vi "Auto State Machine.vi"   [LabVIEW 2013]
uses:
  typedefs/fg_typedef.ctl
  typedefs/State Machine/singleUseSubstate.ctl
  typedefs/State Machine/subStates.ctl
  typedefs/DevRef Type.ctl
  typedefs/Vision/vision enable.ctl
panel:
  # "A State Machine to Handle One or Two Ball Autonomous"
types:
  T1 = typedef "fg_typedef.ctl" = enum16{"Get", "Set"}
  T2 = typedef "subStates.ctl" = enum16{"null", "wait", "driver control", "auto", "manual override", "hold position", "rotate", "pickup", "pass", "recover pass", "load", "goto shoot", "shoot high goal", "shoot low goal", "cancel arm", "cancel shooter", "end", "test"}
  T3 = typedef "singleUseSubstate.ctl" = enum16{"null", "wait", "shift high", "shift low", "extend shooter", "retract shooter", "latch", "unlatch", "end"}
  T4 = typedef "vision enable.ctl" = enum16{"Enable", "Disable", "Stop"}
  T5 = typedef "DevRef Type.ctl" = enum16{"Shooter Solenoid", "Latch Solenoid", "Right Up Sensor", "Right Down Sensor", "Hold Sensor", "Arm Encoder"}
  T6 = typedef "WPI_EncoderDevRef.ctl" = cluster{"DevStatus":errorcluster, "EncoderIndex":T7, "CounterIndex":T8, "DistancePerCount":dbl, "Decoding Type":T9}
  T7 = typedef "FPGA_EncoderIdx.ctl" = enum8{"Enc 0", "Enc 1", "Enc 2", "Enc 3", "Invalid"}
  T8 = typedef "FPGA_CounterCtrSystemIndex.ctl" = enum8{"Ctr 0", "Ctr 1", "Ctr 2", "Ctr 3", "Ctr 4", "Ctr 5", "Ctr 6", "Ctr 7", "Invalid"}
  T9 = typedef "WPI_EncoderType.ctl" = enum16{"1x", "2x", "4x"}
  T10 = typedef "vision data.ctl" = cluster{"x":dbl, "y":dbl, "area":dbl, "width":dbl, "height":dbl, "Hot Goal Present?":bool, "distance":dbl}
  T11 = typedef "WPI_DigitalInputDevRef.ctl" = cluster{"DevStatus":errorcluster, "DIO Channel":T12, "Digital Module":T13}
  T12 = typedef "FPGA_DIOChannel.ctl" = enum8{"DIO 1", "DIO 2", "DIO 3", "DIO 4", "DIO 5", "DIO 6", "DIO 7", "DIO 8", "DIO 9", "DIO 10", "DIO 11", "DIO 12", "DIO 13", "DIO 14", "Invalid"}
  T13 = typedef "FPGA_TypedefDigitalModule.ctl" = enum16{"Digital Module 1", "Digital Module 2"}
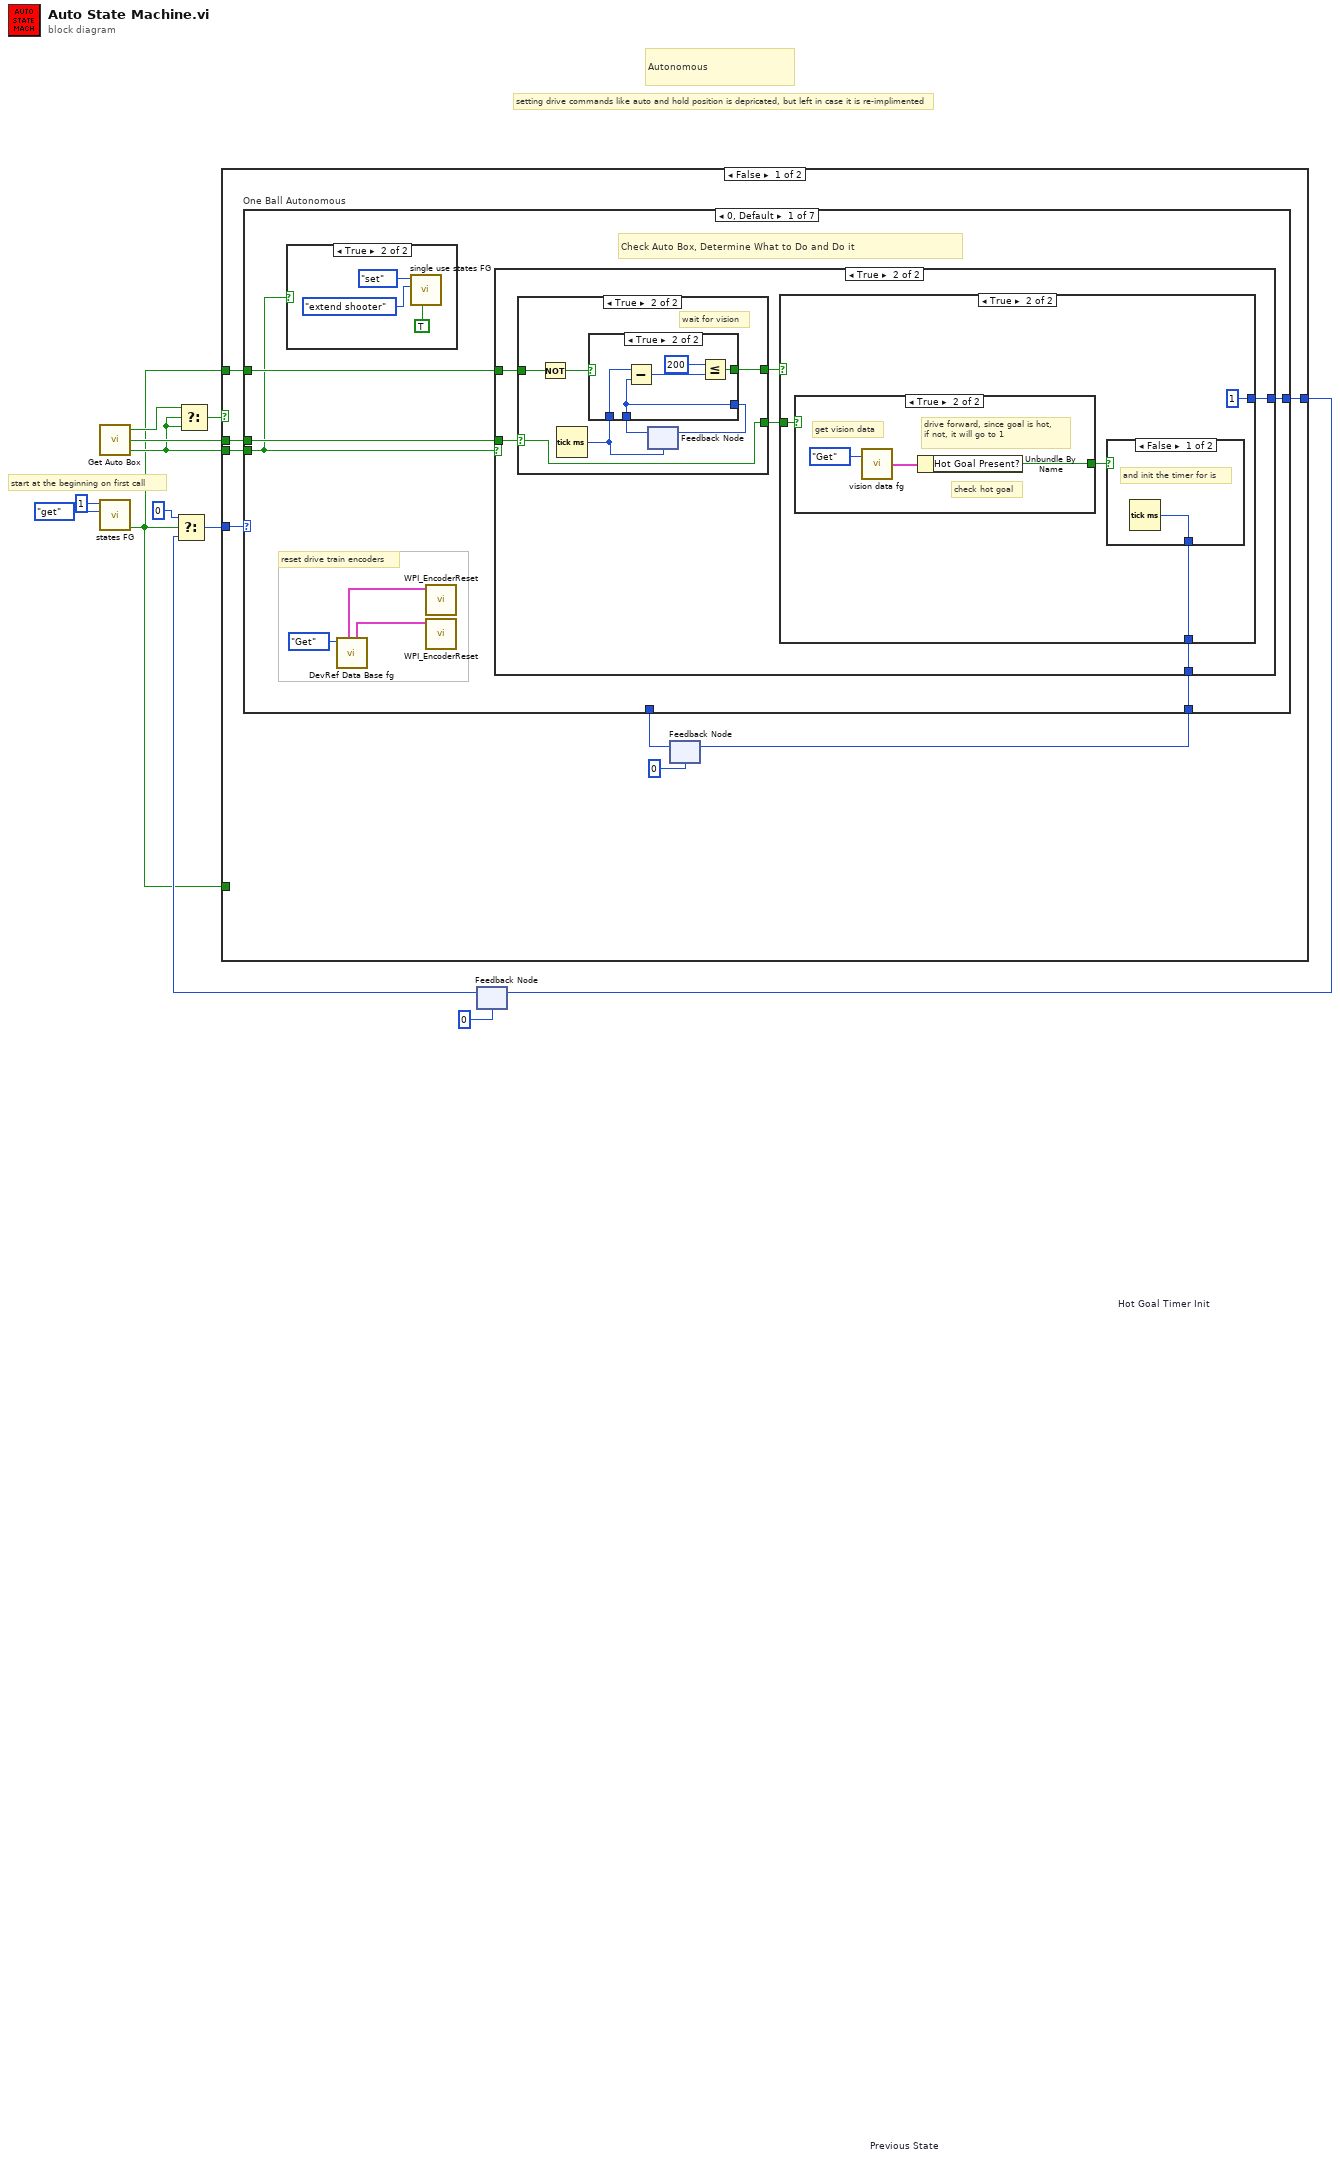
[diagram p0: block diagram]
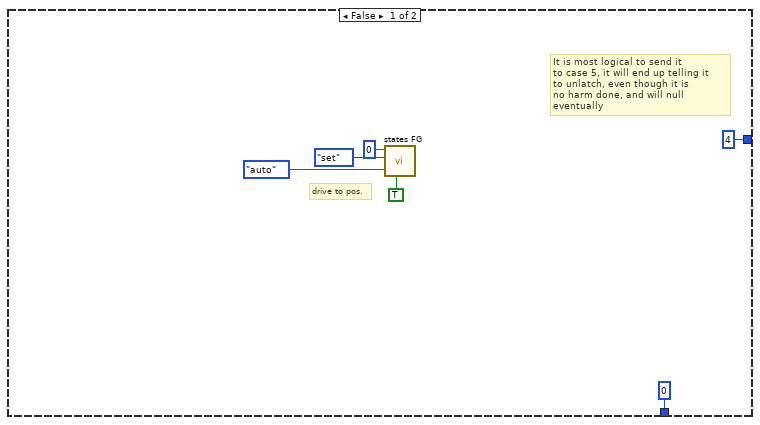
[diagram p2: hidden frame]
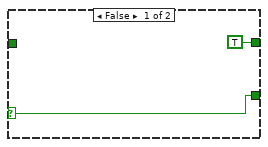
[diagram p3: hidden frame]
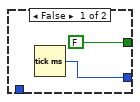
[diagram p4: hidden frame]
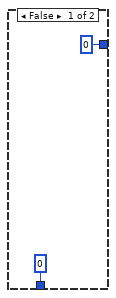
[diagram p5: hidden frame]
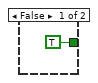
[diagram p6: hidden frame]
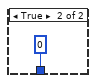
[diagram p7: hidden frame]
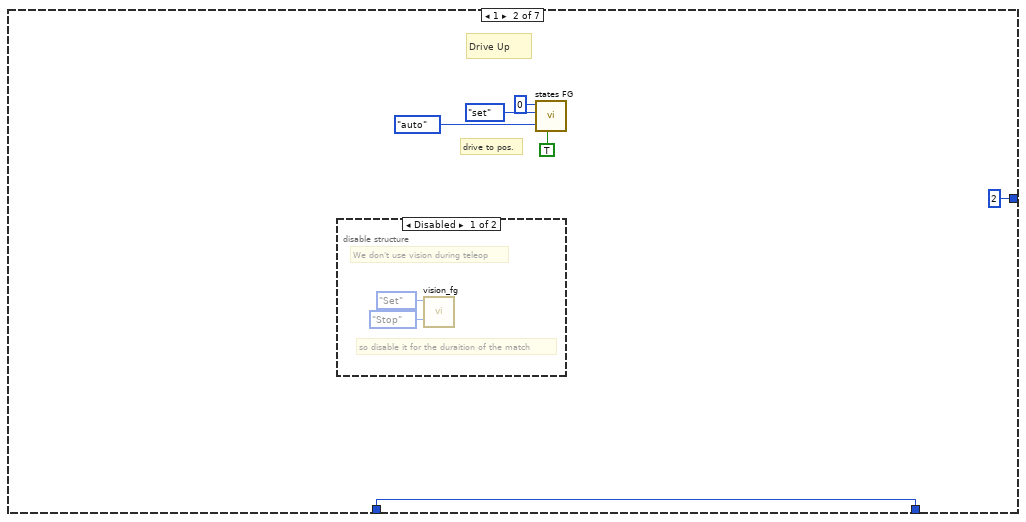
[diagram p9: hidden frame]
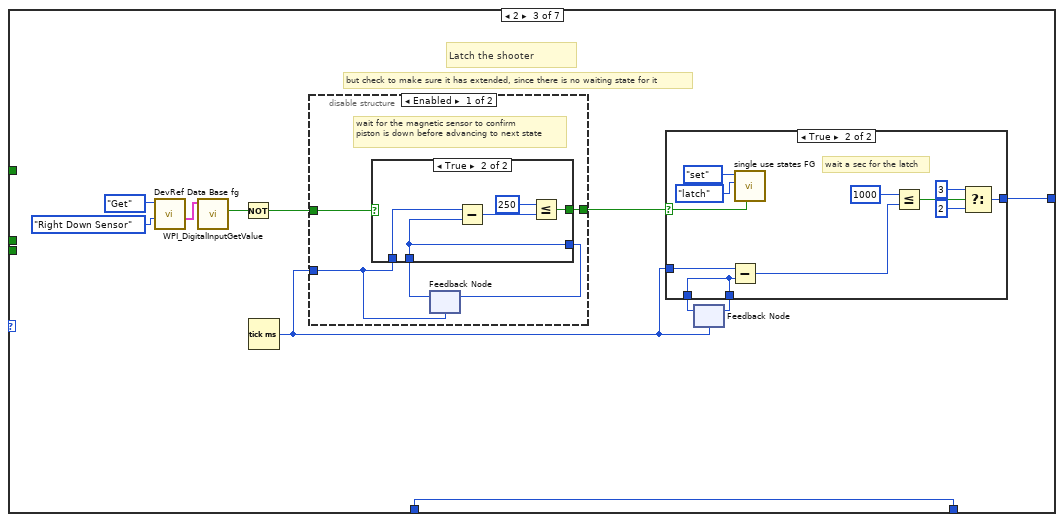
[diagram p11: hidden frame]
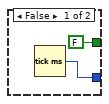
[diagram p12: hidden frame]
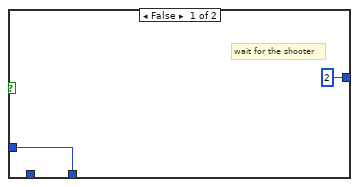
[diagram p14: hidden frame]
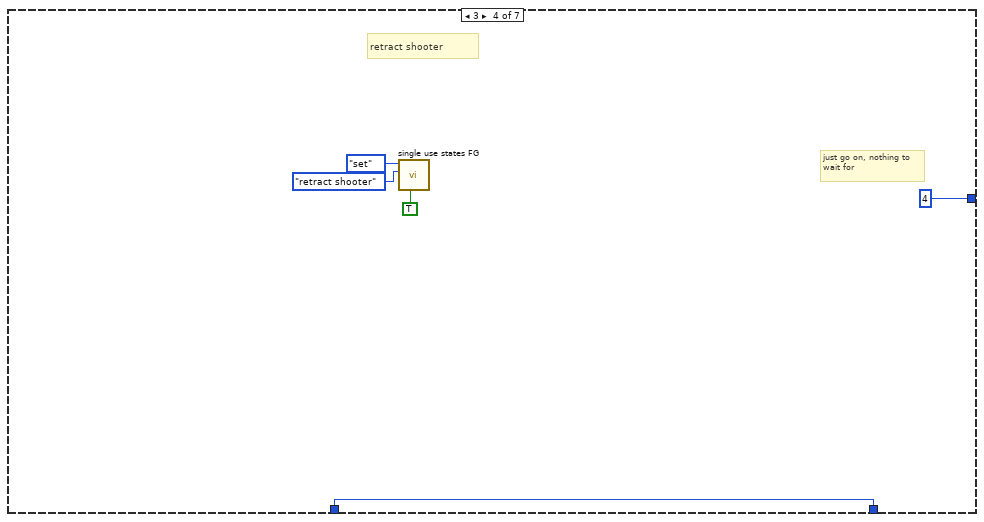
[diagram p15: hidden frame]
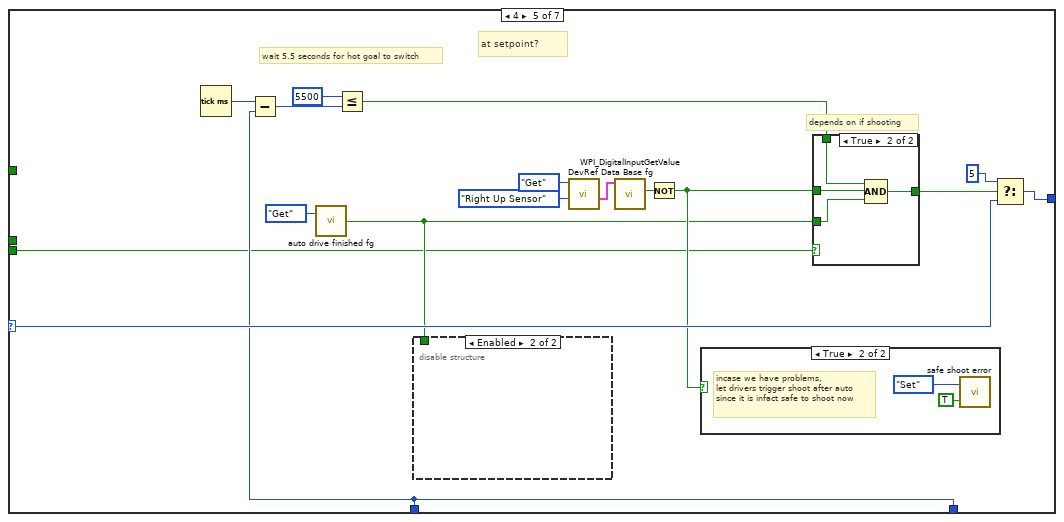
[diagram p16: hidden frame]
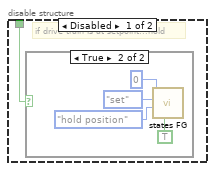
[diagram p18: hidden frame]
diagram:
  # "setting drive commands like auto and hold position is depricated, but left in case it is re-implimented"
  # "start at the beginning on first call"
  # "Autonomous"
  n1 = call "Get Auto Box.vi"() -> ("Shoot During Autonomous?"=w2:bool, "Use Hot Goal?"=w5:bool, "2 Ball Autonomous?"=w3:bool)
  n2 = call "states FG.vi"("menu (get)"=enum16{"set", "get"}."get", "Loop ID"=1) -> ("first call?"=w1:bool)  [unwired: 6 in, 3 out]
  n3 = Select(t=w3, s=w2, f=w2) -> (s? t:f=w4:bool)
  n4 = feedback #1 "Previous State"(u8 0) -> (w8:u8)
  n5 = Select(t=u8 0, s=w1, f=w8) -> (s? t:f=w10:u8)
  n6 = case shown="False" w4 {
    tunnel: w10 -> [w20 w186]
    tunnel: [w19 w179] -> w6
    tunnel: w1 -> [w16 _]
    tunnel: w2 -> [w15 _]
    tunnel: w5 -> [w14 _]
    tunnel: w1 -> [_ w183]
    frame False {
      n7 = feedback #2 "Hot Goal Timer Init"(u32 0 ("millisecond timer value")) -> (w17:u32)
      n8 = case "One Ball Autonomous" shown="0, Default" w20 {
        selector: w20 -> [_ _ _ _ w138 _ w175]
        tunnel: [w28 u8 2 ("t") w86 u8 4 ("t") w136 u8 6 ("t") w175] -> w19
        tunnel: w17 -> [_ w77 w80 w117 w127 w151 w158]
        tunnel: w16 -> [w24 _ _ _ _ _ _]
        tunnel: w15 -> [w22 _ _ _ w122 _ _]
        tunnel: w14 -> [w23 _ _ _ _ _ _]
        tunnel: [w21 w77 w80 w117 w127 w151 w158] -> w13
        frame 0, Default {
          # "reset drive train encoders"
          # "Check Auto Box, Determine What to Do and Do it"
          n9 = case shown="True" w22 {
            frame False {
            }
            frame True {
              n10 = call "single use states FG.vi"("exit in"=TRUE, "substate"=singleUseSubstate."extend shooter", "menu (get)"=enum16{"set", "get"}."set") -> ()  [unwired: 5 in, 4 out]
            }
          }
          n11 = call "DevRef Data Base fg.vi"("Menu"=fg_typedef."Get") -> ("right drive encoder"=w25:T6, "left drive encoder"=w26:T6)  [unwired: 2 in, 7 out]
          n12 = call <vilib>:"WPI_EncoderReset.vi"("EncoderDevRef"=w26) -> ()  [unwired: 9 in, 2 out]
          n13 = call <vilib>:"WPI_EncoderReset.vi"("EncoderDevRef"=w25) -> ()  [unwired: 9 in, 2 out]
          n14 = case shown="True" w22 {
            tunnel: [u8 4 ("f") w40] -> w28
            tunnel: w24 -> [_ w39]
            tunnel: w23 -> [_ w37]
            tunnel: [u32 0 ("millisecond timer value") w35] -> w21
            frame False {
              # "It is most logical to send it\nto case 5, it will end up telling it\nto unlatch, even though it is\nno harm done, and will null eventually"
              # "drive to pos."
              n15 = call "states FG.vi"("exit in"=TRUE, "subState in"=subStates."auto", "menu (get)"=enum16{"set", "get"}."set", "Loop ID"=0) -> ()  [unwired: 4 in, 4 out]
            }
            frame True {
              n16 = case shown="True" w37 {
                selector: w37 -> [w41 w43]
                tunnel: w39 -> [_ w49]
                tunnel: [TRUE w48] -> w38
                tunnel: [w41 w43] -> w36
                frame False {
                }
                frame True {
                  # "wait for vision"
                  n17 = Not(x=w49) -> (.not. x?=w44:bool)
                  n18 = Tick Count (ms)() -> (millisecond timer value=w47:u32)
                  n19 = feedback #3(w47) -> (w45:u32)
                  n20 = case shown="True" w44 {
                    tunnel: w47 -> [_ w54]
                    tunnel: [w51 w52] -> w46
                    tunnel: w45 -> [_ w52]
                    tunnel: [FALSE w53] -> w48
                    frame False {
                      n21 = Tick Count (ms)() -> (millisecond timer value=w51:u32)
                    }
                    frame True {
                      n22 = Subtract(x=w54, y=w52) -> (x-y=w56:u32)
                      n23 = Less Or Equal?(x=u32 200, y=w56) -> (x <= y?=w53:bool)
                    }
                  }
                  n24 = feedback-in #3(w46) -> ()
                }
              }
              n25 = case shown="True" w38 {
                tunnel: [u8 0 ("f") u8 1 ("f")] -> w40
                tunnel: w36 -> [_ w61]
                tunnel: [u32 0 ("millisecond timer value") w59] -> w35
                frame False {
                }
                frame True {
                  n26 = case shown="True" w61 {
                    tunnel: [TRUE ("Hot Goal Present?") w66] -> w62
                    frame False {
                    }
                    frame True {
                      # "drive forward, since goal is hot,\nif not, it will go to 1"
                      # "check hot goal"
                      # "get vision data"
                      n27 = call "vision data fg.vi"("Menu"=fg_typedef."Get") -> ("Output"=w64:T10)  [unwired: 1 in]
                      n28 = Unbundle By Name(w64) -> ("Hot Goal Present?"=w66:bool)
                    }
                  }
                  n29 = case shown="False" w62 {
                    tunnel: [w67 u32 0 ("millisecond timer value")] -> w59
                    frame False {
                      # "and init the timer for is"
                      n30 = Tick Count (ms)() -> (millisecond timer value=w67:u32)
                    }
                    frame True {
                    }
                  }
                }
              }
            }
          }
        }
        frame 1 {
          # "drive to pos."
          # "Drive Up"
          n31 = disable-structure shown="Disabled" {
            frame Disabled {
              # "so disable it for the duraition of the match"
              # "We don't use vision during teleop"
              n32 = call "vision_fg.vi"("Action"=vision_enable."Stop", "Menu"=fg_typedef."Set" ("Enum")) -> ()  [unwired: 1 in, 2 out]
            }
            frame Enabled {
            }
          }
          n33 = call "states FG.vi"("exit in"=TRUE, "subState in"=subStates."auto", "menu (get)"=enum16{"set", "get"}."set", "Loop ID"=0) -> ()  [unwired: 4 in, 4 out]
        }
        frame 2 {
          # "but check to make sure it has extended, since there is no waiting state for it"
          # "Latch the shooter"
          n34 = call "DevRef Data Base fg.vi"("DevRef to Get"=DevRef_Type."Right Down Sensor", "Menu"=fg_typedef."Get") -> ("Selected Sensor"=w90:T11)  [unwired: 1 in, 8 out]
          n35 = call <vilib>:"WPI_DigitalInputGetValue.vi"("DigitalInputDevRef"=w90) -> ("Value"=w89:bool)  [unwired: 8 in, 2 out]
          n36 = Not(x=w89) -> (.not. x?=w83:bool)
          n37 = Tick Count (ms)() -> (millisecond timer value=w82:u32)
          n38 = disable-structure shown="Enabled" {
            disable-tunnel: w83 -> [w95 w103]
            disable-tunnel: [w92 w103] -> w81
            disable-tunnel: w82 -> [w91 _]
            frame Enabled {
              # "wait for the magnetic sensor to confirm \npiston is down before advancing to next state"
              n39 = feedback #4(w91) -> (w93:u32)
              n40 = case shown="True" w95 {
                tunnel: w91 -> [_ w100]
                tunnel: [w97 w98] -> w94
                tunnel: w93 -> [_ w98]
                tunnel: [FALSE w99] -> w92
                frame False {
                  n41 = Tick Count (ms)() -> (millisecond timer value=w97:u32)
                }
                frame True {
                  n42 = Subtract(x=w100, y=w98) -> (x-y=w102:u32)
                  n43 = Less Or Equal?(x=u32 250, y=w102) -> (x <= y?=w99:bool)
                }
              }
              n44 = feedback-in #4(w94) -> ()
            }
            frame Disabled {
            }
          }
          n45 = feedback #5(w82) -> (w87:u32)
          n46 = case shown="True" w81 {
            selector: w81 -> [_ w112]
            tunnel: [w104 w114] -> w88
            tunnel: w87 -> [_ w114]
            tunnel: w82 -> [w104 w113]
            tunnel: [u8 2 ("f") w107] -> w86
            frame False {
              # "wait for the shooter"
            }
            frame True {
              # "wait a sec for the latch"
              n47 = Subtract(x=w113, y=w114) -> (x-y=w109:u32)
              n48 = call "single use states FG.vi"("exit in"=w112, "substate"=singleUseSubstate."latch", "menu (get)"=enum16{"set", "get"}."set") -> ()  [unwired: 5 in, 4 out]
              n49 = Less Or Equal?(x=u32 1000, y=w109) -> (x <= y?=w106:bool)
              n50 = Select(t=u8 3, s=w106, f=u8 2) -> (s? t:f=w107:u8)
            }
          }
          n51 = feedback-in #5(w88) -> ()
        }
        frame 3 {
          # "just go on, nothing to\nwait for"
          # "retract shooter"
          n52 = call "single use states FG.vi"("exit in"=TRUE, "substate"=singleUseSubstate."retract shooter", "menu (get)"=enum16{"set", "get"}."set") -> ()  [unwired: 5 in, 4 out]
        }
        frame 4 {
          # "depends on if shooting"
          # "wait 5.5 seconds for hot goal to switch"
          # "at setpoint?"
          n53 = Tick Count (ms)() -> (millisecond timer value=w128:u32)
          n54 = Subtract(x=w128, y=w127) -> (x-y=w130:u32)
          n55 = call "auto drive finished fg.vi"("Menu"=fg_typedef."Get") -> ("Done"=w124:bool)  [unwired: 1 in]
          n56 = Less Or Equal?(x=u32 5500, y=w130) -> (x <= y?=w126:bool)
          n57 = disable-structure shown="Enabled" {
            disable-tunnel: w124 -> [w144 _]
            frame Disabled {
              # "if drive train is at setpoint...hold"
              n58 = case shown="True" w144 {
                frame False {
                }
                frame True {
                  n59 = call "states FG.vi"("exit in"=TRUE, "subState in"=subStates."hold position" ("y"), "menu (get)"=enum16{"set", "get"}."set", "Loop ID"=0) -> ()  [unwired: 4 in, 4 out]
                }
              }
            }
            frame Enabled {
            }
          }
          n60 = call "DevRef Data Base fg.vi"("DevRef to Get"=DevRef_Type."Right Up Sensor", "Menu"=fg_typedef."Get") -> ("Selected Sensor"=w135:T11)  [unwired: 1 in, 8 out]
          n61 = call <vilib>:"WPI_DigitalInputGetValue.vi"("DigitalInputDevRef"=w135) -> ("Value"=w134:bool)  [unwired: 8 in, 2 out]
          n62 = Not(x=w134) -> (.not. x?=w125:bool)
          n63 = case shown="True" w125 {
            frame False {
            }
            frame True {
              # "incase we have problems,\nlet drivers trigger shoot after auto\nsince it is infact safe to shoot now"
              n64 = call "safe shoot error.vi"("Can Shoot Safely?"=TRUE, "Menu"=fg_typedef."Set") -> ()  [unwired: 1 out]
            }
          }
          n65 = case shown="True" w122 {
            tunnel: w126 -> [_ w143]
            tunnel: w125 -> [_ w142]
            tunnel: w124 -> [w139 w141]
            tunnel: [w139 w140] -> w123
            frame False {
            }
            frame True {
              n66 = Compound Arithmetic op=AND(w143, w142, w141) -> (w140:bool)
            }
          }
          n67 = Select(t=u8 5, s=w123, f=w138) -> (s? t:f=w136:u8)
        }
        frame 5 {
          w154 = FALSE ("Can Shoot Safely?")
          w153 = fg_typedef."Set" ("Menu")
          # "unlatch shooter"
          # "SHOOT!!!"
          n68 = call "safe shoot error.vi"("Can Shoot Safely?"=w154, "Menu"=w153) -> ()  [unwired: 1 out]
          n69 = call "auto drive finished fg.vi"("Done?"=w154, "Menu"=w153) -> ()  [unwired: 1 out]
          n70 = call "single use states FG.vi"("exit in"=TRUE, "substate"=singleUseSubstate."unlatch", "menu (get)"=enum16{"set", "get"}."set") -> ()  [unwired: 5 in, 4 out]
        }
        frame 6 {
          # "null things"
          # "null all the things"
          n71 = call "states FG.vi"("exit in"=TRUE, "subState in"=subStates."null", "menu (get)"=enum16{"set", "get"}."set", "Loop ID"=0) -> ()  [unwired: 4 in, 4 out]
          n72 = call "states FG.vi"("exit in"=TRUE, "subState in"=subStates."null", "menu (get)"=enum16{"set", "get"}."set", "Loop ID"=1) -> ()  [unwired: 4 in, 4 out]
          n73 = call "states FG.vi"("exit in"=TRUE, "subState in"=subStates."null", "menu (get)"=enum16{"set", "get"}."set", "Loop ID"=2) -> ()  [unwired: 4 in, 4 out]
          n74 = call "states FG.vi"("exit in"=TRUE, "subState in"=subStates."null", "menu (get)"=enum16{"set", "get"}."set", "Loop ID"=3) -> ()  [unwired: 4 in, 4 out]
        }
      }
      n75 = feedback-in #2(w13) -> ()
    }
    frame True {
      n76 = feedback #6 "Wait Timer Init"(u32 0 ("millisecond timer value")) -> (w176:u32)
      n77 = case "Two Ball Autonomous" shown="0, Default" w186 {
        selector: w186 -> [_ w258 _ w277 _ w311 _ _ w332 w370 _ w388]
        tunnel: [u8 1 ("t") w260 u8 3 ("t") w274 u8 5 ("t") w313 u8 7 ("t") u8 8 ("t") w333 w369 u8 11 ("t") w388] -> w179
        tunnel: [_ _ w268 w275 _ _ _ _ _ _ _ _] -> w177
        tunnel: w176 -> [_ _ _ w276 _ _ _ _ _ _ _ _]
        frame 0, Default {
          # "full reverse is belts in"
          # "belts on"
          # "up setpoint"
          # "put arm out"
          # "Arm Up, Belts In"
          # "reset drive train encoders"
          n78 = call "DevRef Data Base fg.vi"("Menu"=fg_typedef."Get") -> ("right drive encoder"=w255:T6, "left drive encoder"=w256:T6)  [unwired: 2 in, 7 out]
          n79 = call <vilib>:"WPI_EncoderReset.vi"("EncoderDevRef"=w256) -> ()  [unwired: 9 in, 2 out]
          n80 = call <vilib>:"WPI_EncoderReset.vi"("EncoderDevRef"=w255) -> ()  [unwired: 9 in, 2 out]
          n81 = call "Arm Setpoint FG.vi"("Setpoint In"=55.0, "Menu"=fg_typedef."Set") -> ()  [unwired: 1 out]
          n82 = call "states FG.vi"("exit in"=TRUE, "subState in"=subStates."auto", "menu (get)"=enum16{"set", "get"}."set", "Loop ID"=3) -> ()  [unwired: 4 in, 4 out]
          n83 = call "Belt Speed FG.vi"("Speed In"=-1.0 ("Setpoint In"), "Menu"=fg_typedef."Set") -> ()  [unwired: 1 out]
          n84 = call "states FG.vi"("exit in"=TRUE, "subState in"=subStates."auto", "menu (get)"=enum16{"set", "get"}."set", "Loop ID"=2) -> ()  [unwired: 4 in, 4 out]
        }
        frame 1 {
          # "Wait for Arm"
          n85 = call "DevRef Data Base fg.vi"("DevRef to Get"=DevRef_Type."Arm Encoder", "Menu"=fg_typedef."Get") -> ("Selected Encoder"=w267:T6)  [unwired: 1 in, 8 out]
          n86 = call <vilib>:"WPI_EncoderGet.vi"("EncoderDevRef"=w267) -> ("Distance"=w266:dbl)  [unwired: 5 in, 5 out]
          n87 = In Range and Coerce(upper limit=55.0, x=w266, lower limit=45.0) -> (In Range?=w259:bool)  [unwired: 1 out]
          n88 = Select(t=u8 2, s=w259, f=w258) -> (s? t:f=w260:u8)
        }
        frame 2 {
          # "drive to reverse position"
          n89 = Tick Count (ms)() -> (millisecond timer value=w268:u32)
          n90 = call "states FG.vi"("exit in"=TRUE, "subState in"=subStates."auto", "menu (get)"=enum16{"set", "get"}."set", "Loop ID"=0) -> ()  [unwired: 4 in, 4 out]
        }
        frame 3 {
          # "Wait for Ball"
          n91 = disable-structure shown="Enabled" {
            disable-tunnel: w277 -> [w279 w288]
            disable-tunnel: w276 -> [_ w290]
            disable-tunnel: [_ w290] -> w275
            disable-tunnel: [w278 w286] -> w274
            frame Disabled {
              n92 = call "DevRef Data Base fg.vi"("DevRef to Get"=DevRef_Type."Hold Sensor", "Menu"=fg_typedef."Get") -> ("Selected Sensor"=w283:T11)  [unwired: 1 in, 8 out]
              n93 = call <vilib>:"WPI_DigitalInputGetValue.vi"("DigitalInputDevRef"=w283) -> ("Value"=w285:bool)  [unwired: 8 in, 2 out]
              n94 = Not(x=w285) -> (.not. x?=w284:bool)
              n95 = Select(t=u8 4, s=w284, f=w279) -> (s? t:f=w278:u8)
            }
            frame Enabled {
              n96 = Tick Count (ms)() -> (millisecond timer value=w293:u32)
              n97 = Subtract(x=w293, y=w290) -> (x-y=w292:u32)
              n98 = Less Or Equal?(x=u32 1000, y=w292) -> (x <= y?=w289:bool)
              n99 = Select(t=u8 4, s=w289, f=w288) -> (s? t:f=w286:u8)
            }
          }
        }
        frame 4 {
          # "drive to forward position"
          # "arm rests on ball"
          # "reset fg"
          # "reset fg"
          # "Belts Off, Arm Hold Ball"
          n100 = call "states FG.vi"("exit in"=TRUE, "subState in"=subStates."auto", "menu (get)"=enum16{"set", "get"}."set", "Loop ID"=0) -> ()  [unwired: 4 in, 4 out]
          n101 = call "Belt Speed FG.vi"("Speed In"=0.0 ("Setpoint In"), "Menu"=fg_typedef."Set") -> ()  [unwired: 1 out]
          n102 = call "states FG.vi"("exit in"=TRUE, "subState in"=subStates."null", "menu (get)"=enum16{"set", "get"}."set", "Loop ID"=3) -> ()  [unwired: 4 in, 4 out]
          n103 = call "states FG.vi"("exit in"=TRUE, "subState in"=subStates."null", "menu (get)"=enum16{"set", "get"}."set", "Loop ID"=2) -> ()  [unwired: 4 in, 4 out]
          n104 = call "Arm Setpoint FG.vi"("Setpoint In"=0.0, "Menu"=fg_typedef."Set") -> ()  [unwired: 1 out]
        }
        frame 5 {
          w317 = fg_typedef."Get" ("Menu")
          # "Ready to Shoot 1st Ball?"
          n105 = call "safe shoot error.vi"("Menu"=w317) -> ("Can Shoot Safely?"=w316:bool)  [unwired: 1 in]
          n106 = call "auto drive finished fg.vi"("Menu"=w317) -> ("Done"=w315:bool)  [unwired: 1 in]
          n107 = And(x=w316, y=w315) -> (x .and. y?=w312:bool)
          n108 = Select(t=u8 6, s=w312, f=w311) -> (s? t:f=w313:u8)
        }
        frame 6 {
          w320 = FALSE ("Can Shoot Safely?")
          w319 = fg_typedef."Set" ("Menu")
          # "unlatch shooter"
          # "stop driving"
          n109 = call "states FG.vi"("exit in"=TRUE, "subState in"=subStates."hold position", "menu (get)"=enum16{"set", "get"}."set", "Loop ID"=0) -> ()  [unwired: 4 in, 4 out]
          n110 = call "safe shoot error.vi"("Can Shoot Safely?"=w320, "Menu"=w319) -> ()  [unwired: 1 out]
          n111 = call "auto drive finished fg.vi"("Done?"=w320, "Menu"=w319) -> ()  [unwired: 1 out]
          n112 = call "single use states FG.vi"("exit in"=TRUE, "substate"=singleUseSubstate."unlatch", "menu (get)"=enum16{"set", "get"}."set") -> ()  [unwired: 5 in, 4 out]
        }
        frame 7 {
          # "Cock again"
          # "extend shooter"
          n113 = call "single use states FG.vi"("exit in"=TRUE, "substate"=singleUseSubstate."extend shooter", "menu (get)"=enum16{"set", "get"}."set") -> ()  [unwired: 5 in, 4 out]
        }
        frame 8 {
          # "Wait to Latch Shooter, Then Latch"
          n114 = call "DevRef Data Base fg.vi"("DevRef to Get"=DevRef_Type."Right Down Sensor", "Menu"=fg_typedef."Get") -> ("Selected Sensor"=w335:T11)  [unwired: 1 in, 8 out]
          n115 = call <vilib>:"WPI_DigitalInputGetValue.vi"("DigitalInputDevRef"=w335) -> ("Value"=w334:bool)  [unwired: 8 in, 2 out]
          n116 = Tick Count (ms)() -> (millisecond timer value=w342:u32)
          n117 = Not(x=w334) -> (.not. x?=w338:bool)
          n118 = disable-structure shown="Enabled" {
            disable-tunnel: w338 -> [w360 w368]
            disable-tunnel: [w357 w368] -> w341
            disable-tunnel: w342 -> [w356 _]
            frame Enabled {
              # "wait for the magnetic sensor to confirm \npiston is down before advancing to next state"
              n119 = feedback #7(w356) -> (w358:u32)
              n120 = case shown="True" w360 {
                tunnel: w356 -> [_ w365]
                tunnel: [w362 w363] -> w359
                tunnel: w358 -> [_ w363]
                tunnel: [FALSE w364] -> w357
                frame False {
                  n121 = Tick Count (ms)() -> (millisecond timer value=w362:u32)
                }
                frame True {
                  n122 = Subtract(x=w365, y=w363) -> (x-y=w367:u32)
                  n123 = Less Or Equal?(x=u32 250, y=w367) -> (x <= y?=w364:bool)
                }
              }
              n124 = feedback-in #7(w359) -> ()
            }
            frame Disabled {
            }
          }
          n125 = feedback #8(w342) -> (w340:u32)
          n126 = case shown="True" w341 {
            selector: w341 -> [_ w351]
            tunnel: [w344 w353] -> w339
            tunnel: w340 -> [_ w353]
            tunnel: w342 -> [w344 w352]
            tunnel: [w343 w347] -> w333
            tunnel: w332 -> [w343 w345]
            frame False {
              # "wait for the shooter"
            }
            frame True {
              # "wait a sec for the latch"
              n127 = Subtract(x=w352, y=w353) -> (x-y=w348:u32)
              n128 = call "single use states FG.vi"("exit in"=w351, "substate"=singleUseSubstate."latch", "menu (get)"=enum16{"set", "get"}."set") -> ()  [unwired: 5 in, 4 out]
              n129 = Less Or Equal?(x=u32 1000, y=w348) -> (x <= y?=w346:bool)
              n130 = Select(t=u8 9, s=w346, f=w345) -> (s? t:f=w347:u8)
            }
          }
          n131 = feedback-in #8(w339) -> ()
        }
        frame 9 {
          # "Retract Shooter"
          # "retract shooter"
          n132 = call "single use states FG.vi"("exit in"=TRUE, "substate"=singleUseSubstate."retract shooter", "menu (get)"=enum16{"set", "get"}."set") -> ()  [unwired: 5 in, 4 out]
          n133 = call "DevRef Data Base fg.vi"("DevRef to Get"=DevRef_Type."Right Up Sensor", "Menu"=fg_typedef."Get") -> ("Selected Sensor"=w371:T11)  [unwired: 1 in, 8 out]
          n134 = call <vilib>:"WPI_DigitalInputGetValue.vi"("DigitalInputDevRef"=w371) -> ("Value"=w372:bool)  [unwired: 8 in, 2 out]
          n135 = Not(x=w372) -> (.not. x?=w376:bool)
          n136 = case shown="True" w376 {
            frame False {
            }
            frame True {
              # "incase we have problems,\nlet drivers trigger shoot after auto\nsince it is infact safe to shoot now"
              n137 = call "safe shoot error.vi"("Can Shoot Safely?"=TRUE, "Menu"=fg_typedef."Set") -> ()  [unwired: 1 out]
            }
          }
          n138 = Select(t=u8 10, s=w376, f=w370) -> (s? t:f=w369:u8)
        }
        frame 10 {
          w384 = FALSE ("Can Shoot Safely?")
          w383 = fg_typedef."Set" ("Menu")
          # "unlatch shooter"
          # "Shoot Second Ball"
          n139 = call "safe shoot error.vi"("Can Shoot Safely?"=w384, "Menu"=w383) -> ()  [unwired: 1 out]
          n140 = call "auto drive finished fg.vi"("Done?"=w384, "Menu"=w383) -> ()  [unwired: 1 out]
          n141 = call "single use states FG.vi"("exit in"=TRUE, "substate"=singleUseSubstate."unlatch", "menu (get)"=enum16{"set", "get"}."set") -> ()  [unwired: 5 in, 4 out]
        }
        frame 11 {
          # "Null Everything"
          # "null things"
          n142 = call "states FG.vi"("exit in"=TRUE, "subState in"=subStates."null", "menu (get)"=enum16{"set", "get"}."set", "Loop ID"=0) -> ()  [unwired: 4 in, 4 out]
          n143 = call "states FG.vi"("exit in"=TRUE, "subState in"=subStates."null", "menu (get)"=enum16{"set", "get"}."set", "Loop ID"=1) -> ()  [unwired: 4 in, 4 out]
          n144 = call "states FG.vi"("exit in"=TRUE, "subState in"=subStates."null", "menu (get)"=enum16{"set", "get"}."set", "Loop ID"=2) -> ()  [unwired: 4 in, 4 out]
          n145 = call "states FG.vi"("exit in"=TRUE, "subState in"=subStates."null", "menu (get)"=enum16{"set", "get"}."set", "Loop ID"=3) -> ()  [unwired: 4 in, 4 out]
        }
      }
      n146 = feedback-in #6(w177) -> ()
      n147 = feedback #9 "Previous State"(u8 0) -> (w181:u8)
      n148 = Select(t=u8 0, s=w183, f=w181) -> (s? t:f=w184:u8)
      n149 = case "Parallel Initial Pneumatics" shown="0, Default" w184 {
        selector: w184 -> [_ w191 w238 w241]
        tunnel: [u8 1 ("t") w194 w229 w241] -> w180
        frame 0, Default {
          # "Cock Shooter for Pre-Loaded Ball"
          # "extend shooter"
          n150 = call "single use states FG.vi"("exit in"=TRUE, "substate"=singleUseSubstate."extend shooter", "menu (get)"=enum16{"set", "get"}."set") -> ()  [unwired: 5 in, 4 out]
        }
        frame 1 {
          # "Wait to Latch Shooter, Then Latch"
          n151 = call "DevRef Data Base fg.vi"("DevRef to Get"=DevRef_Type."Right Down Sensor", "Menu"=fg_typedef."Get") -> ("Selected Sensor"=w200:T11)  [unwired: 1 in, 8 out]
          n152 = call <vilib>:"WPI_DigitalInputGetValue.vi"("DigitalInputDevRef"=w200) -> ("Value"=w201:bool)  [unwired: 8 in, 2 out]
          n153 = Tick Count (ms)() -> (millisecond timer value=w192:u32)
          n154 = Not(x=w201) -> (.not. x?=w197:bool)
          n155 = disable-structure shown="Enabled" {
            disable-tunnel: w197 -> [w219 w227]
            disable-tunnel: [w216 w227] -> w193
            disable-tunnel: w192 -> [w215 _]
            frame Enabled {
              # "wait for the magnetic sensor to confirm \npiston is down before advancing to next state"
              n156 = feedback #10(w215) -> (w217:u32)
              n157 = case shown="True" w219 {
                tunnel: w215 -> [_ w224]
                tunnel: [w221 w222] -> w218
                tunnel: w217 -> [_ w222]
                tunnel: [FALSE w223] -> w216
                frame False {
                  n158 = Tick Count (ms)() -> (millisecond timer value=w221:u32)
                }
                frame True {
                  n159 = Subtract(x=w224, y=w222) -> (x-y=w226:u32)
                  n160 = Less Or Equal?(x=u32 250, y=w226) -> (x <= y?=w223:bool)
                }
              }
              n161 = feedback-in #10(w218) -> ()
            }
            frame Disabled {
            }
          }
          n162 = feedback #11(w192) -> (w195:u32)
          n163 = case shown="True" w193 {
            selector: w193 -> [_ w210]
            tunnel: [w203 w212] -> w196
            tunnel: w195 -> [_ w212]
            tunnel: w192 -> [w203 w211]
            tunnel: [w202 w206] -> w194
            tunnel: w191 -> [w202 w204]
            frame False {
              # "wait for the shooter"
            }
            frame True {
              # "wait a sec for the latch"
              n164 = Subtract(x=w211, y=w212) -> (x-y=w207:u32)
              n165 = call "single use states FG.vi"("exit in"=w210, "substate"=singleUseSubstate."latch", "menu (get)"=enum16{"set", "get"}."set") -> ()  [unwired: 5 in, 4 out]
              n166 = Less Or Equal?(x=u32 1000, y=w207) -> (x <= y?=w205:bool)
              n167 = Select(t=u8 2, s=w205, f=w204) -> (s? t:f=w206:u8)
            }
          }
          n168 = feedback-in #11(w196) -> ()
        }
        frame 2 {
          # "retract shooter"
          # "Retract Shooter"
          n169 = call "single use states FG.vi"("exit in"=TRUE, "substate"=singleUseSubstate."retract shooter", "menu (get)"=enum16{"set", "get"}."set") -> ()  [unwired: 5 in, 4 out]
          n170 = call "DevRef Data Base fg.vi"("DevRef to Get"=DevRef_Type."Right Up Sensor", "Menu"=fg_typedef."Get") -> ("Selected Sensor"=w234:T11)  [unwired: 1 in, 8 out]
          n171 = call <vilib>:"WPI_DigitalInputGetValue.vi"("DigitalInputDevRef"=w234) -> ("Value"=w233:bool)  [unwired: 8 in, 2 out]
          n172 = Not(x=w233) -> (.not. x?=w228:bool)
          n173 = case shown="True" w228 {
            frame False {
            }
            frame True {
              # "incase we have problems,\nlet drivers trigger shoot after auto\nsince it is infact safe to shoot now"
              n174 = call "safe shoot error.vi"("Can Shoot Safely?"=TRUE, "Menu"=fg_typedef."Set") -> ()  [unwired: 1 out]
            }
          }
          n175 = Select(t=u8 3, s=w228, f=w238) -> (s? t:f=w229:u8)
        }
        frame 3 {
        }
      }
      n176 = feedback-in #9(w180) -> ()
    }
  }
  n177 = feedback-in #1(w6) -> ()
